vi "host_db_logging.vi"() -> ()   [LabVIEW 2011]
uses:
  Output - Cluster.ctl
  <vilib>/addons/database/Connection.llb/DB Tools Open Connec (Path).vi
  <vilib>/addons/database/NI_Database_API.lvlib
panel:
  out "error in (no error)":errorcluster
  in  "Pfad":path=path "C:/Git/B2G/B2G_db_rz.dsn"
  in  "Interval [ms]":u32=1000 min=100 step=1
  in  "DB Log":bool
  in  "stop":bool
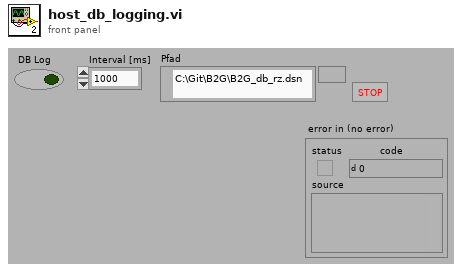
[diagram p1: front panel]
types:
  T1 = typedef "NI_Database_API.lvlib/Conn ObjectReference.ctl" = refnum<k1>
  T2 = typedef "Output - Cluster.ctl" = cluster{"DFS-1 [l]":u64, "FS-3 [l]":dbl, "DFS-1 [l/min]":dbl, "DS-1 [bar]":dbl, "V-10 ZU":bool, "V-14 ZU":bool, "FS-1 [l]":dbl, "FS-2 [l]":dbl, "TS-4 [°C]":dbl, "HS-1":bool, "V-13 [%]":u8, "V-15 [%]":u8, "P-4 [%]":u8, "P-5 [%]":u8, "Dosierung":bool, "MR Max Füllstand":bool, "MR Min Füllstand":bool, "Dosiermenge [l]":sgl, "V-14 AUF":bool, "V-10 AUF":bool, "T-1 Max Füllstand":bool, "T-1 Min Füllstand":bool, "T-2 Max Füllstand":bool, "T-2 Min Füllstand":bool, "pHS-1 [pH]":dbl, "P-4":bool, "P-5":bool, "V-33 AUF":bool, "V-33 ZU":bool, "V-34 AUF":bool, "V-34 ZU":bool}
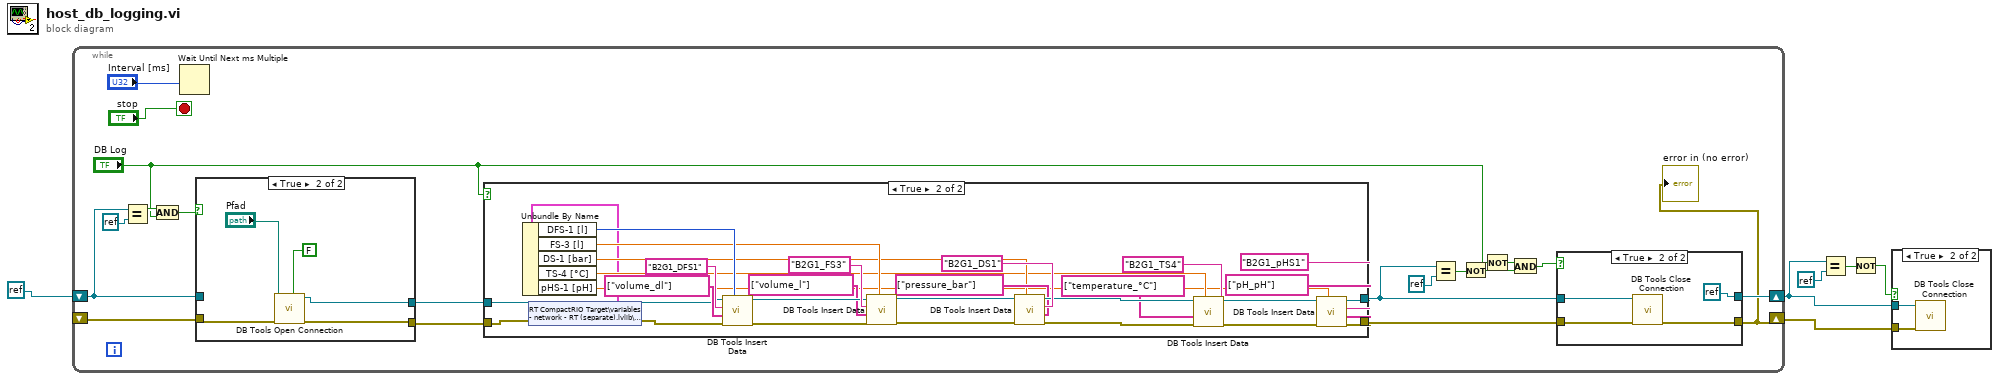
[diagram p0: block diagram]
diagram:
  n1 = while {
    shift-right: [w7] -> w5
    shift-left: _ -> [w21]
    shift-right: [w9] -> w1
    shift-left: refnum<k0> refnum -> [w17]
    stop <- "stop" stop-if-true
    n2 = Equal?(x=w17, y=refnum<k0> refnum) -> (x = y?=w20:bool)
    n3 = And(x=w20, y="DB Log") -> (x .and. y?=w19:bool)
    n4 = Wait Until Next ms Multiple(millisecond multiple="Interval [ms]") -> ()  [unwired: 1 out]
    n5 = case shown="True" w19 {
      tunnel: [w33 w36] -> w23
      tunnel: w17 -> [w33 _]
      tunnel: [w32 w35] -> w22
      tunnel: w21 -> [w32 w34]
      frame False {
      }
      frame True {
        n6 = call-poly <vilib>:"DB Tools Open Connection.vi"("error in (no error)"=w34, "prompt? (F)"=FALSE, "connection information"="Pfad") -> ("error out"=w35:errorcluster, "connection reference"=w36:T1)  [unwired: 5 in]
      }
    }
    n7 = case shown="True" "DB Log" {
      tunnel: [w40 w55] -> w11
      tunnel: [w39 w54] -> w10
      tunnel: w23 -> [w40 w44]
      tunnel: w22 -> [w39 w41]
      frame False {
      }
      frame True {
        n8 = shared-variable "RT CompactRIO Target\\variables - network - RT (separate).lvlib\\data - network"(error in=w41) -> (w43:T2, error out=w42:errorcluster)
        n9 = Unbundle By Name(w43) -> ("DFS-1 [l]"=w53:u64, "FS-3 [l]"=w48:dbl, "DS-1 [bar]"=w47:dbl, "TS-4 [°C]"=w46:dbl, "pHS-1 [pH]"=w45:dbl)
        n10 = call <vilib>:"DB Tools Insert Data.vi"("data"=w53, "error in (no error)"=w42, "columns"=string[] ["volume_dl"], "table"="B2G1_DFS1", "connection reference"=w44) -> ("error out"=w65:errorcluster, "connection reference out"=w66:T1)  [unwired: 5 in]
        n11 = call <vilib>:"DB Tools Insert Data.vi"("data"=w48, "error in (no error)"=w65, "columns"=string[] ["volume_l"], "table"="B2G1_FS3", "connection reference"=w66) -> ("error out"=w63:errorcluster, "connection reference out"=w62:T1)  [unwired: 5 in]
        n12 = call <vilib>:"DB Tools Insert Data.vi"("data"=w47, "error in (no error)"=w63, "columns"=string[] ["pressure_bar"], "table"="B2G1_DS1", "connection reference"=w62) -> ("error out"=w59:errorcluster, "connection reference out"=w60:T1)  [unwired: 5 in]
        n13 = call <vilib>:"DB Tools Insert Data.vi"("data"=w46, "error in (no error)"=w59, "columns"=string[] ["temperature_°C"], "table"="B2G1_TS4", "connection reference"=w60) -> ("error out"=w56:errorcluster, "connection reference out"=w57:T1)  [unwired: 5 in]
        n14 = call <vilib>:"DB Tools Insert Data.vi"("data"=w45, "error in (no error)"=w56, "columns"=string[] ["pH_pH"], "table"="B2G1_pHS1", "connection reference"=w57) -> ("error out"=w54:errorcluster, "connection reference out"=w55:T1)  [unwired: 5 in]
      }
    }
    n15 = Equal?(x=w11, y=refnum<k0> refnum) -> (x = y?=w16:bool)
    n16 = Not(x=w16) -> (.not. x?=w14:bool)
    n17 = Not(x="DB Log") -> (.not. x?=w15:bool)
    n18 = And(x=w15, y=w14) -> (x .and. y?=w8:bool)
    n19 = case shown="True" w8 {
      tunnel: w11 -> [w27 w31]
      tunnel: w10 -> [w26 w30]
      tunnel: [w26 w29] -> w7
      tunnel: [w27 refnum<k0> refnum] -> w9
      frame False {
      }
      frame True {
        n20 = call <vilib>:"DB Tools Close Connection.vi"("error in (no error)"=w30, "connection reference"=w31) -> ("error out"=w29:errorcluster)  [unwired: 5 in]
      }
    }
    "error in (no error)" <- w7
  }
  n21 = Equal?(x=w1, y=refnum<k0> refnum) -> (x = y?=w4:bool)
  n22 = Not(x=w4) -> (.not. x?=w2:bool)
  n23 = case shown="True" w2 {
    tunnel: w5 -> [_ w71]
    tunnel: w1 -> [_ w70]
    frame False {
    }
    frame True {
      n24 = call <vilib>:"DB Tools Close Connection.vi"("error in (no error)"=w71, "connection reference"=w70) -> ()  [unwired: 5 in, 1 out]
    }
  }
